vi "Set Table Column Width.vi"(6 "MeasurementSystem":i32(ring) items=["Default", "US", "Metric"], 8 "error in":errorcluster, 9 "Column Width":dbl format="%.2f", 10 "Number of Columns":i32, 11 "AppendTable":refnum<k7>) -> (0 "error out":errorcluster)   [LabVIEW 2017, in "NI_ReportGenerationCore.lvlib"]
uses:
  <vilib>/Utility/NIReport.llb/NI_ReportGenerationCore.lvlib
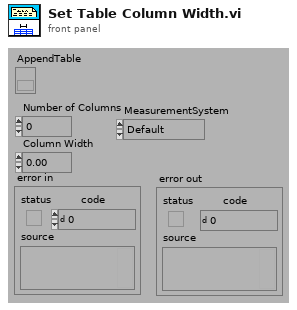
[diagram p1: front panel]
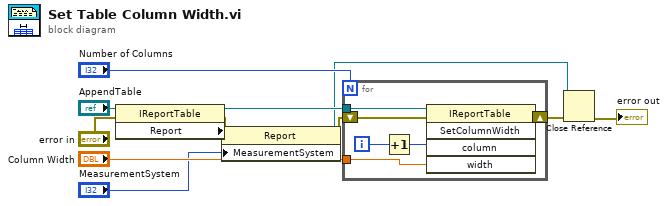
[diagram p0: block diagram]
diagram:
  n1 = property class="IReportTable"(reference="AppendTable", error in="error in") -> (reference out=w6:refnum<k7>, error out=w7:errorcluster, "Report"=w9:refnum<k7>)
  n2 = property class="Report"(reference=w9, error in=w7, "MeasurementSystem"="MeasurementSystem") -> (reference out=w1:refnum<k7>, error out=w8:errorcluster)
  n3 = for {
    N: "Number of Columns" -> [_]
    tunnel: w6 -> [w18]
    tunnel: "Column Width" -> [w17]
    shift-right: [w14] -> w3
    shift-left: w8 -> [w13]
    i -> [w16]
    n4 = Increment(x=w16) -> (x+1=w15:i32)
    n5 = invoke class="IReportTable" method="SetColumnWidth"(reference=w18, error in=w13, "column"=w15, "width"=w17) -> (error out=w14:errorcluster)  [unwired: 1 in, 4 out]
  }
  n6 = Close Reference(reference=w1, error in (no error)=w3) -> (error out=→"error out":errorcluster)
